vi "Verify Bitfile Selection.vi"(5 "Warning text reference":refnum<vi>, 7 "ok button reference in":refnum<vi>, 8 "error in (no error)":errorcluster, 9 "Existing RIO Device Addresses":string[](array[string]), 10 "RIO Device Address":string, 11 "file path":path) -> (0 "error out":errorcluster)   [LabVIEW 2020, in "Engine Simulation Toolkit System Explorer.lvlib"]
uses:
  Engine Simulation Toolkit System Explorer.lvlib
  Shared/Constants and GUIDs.vi
  <userlib>/_OpenG.lib/file/file.llb/File Exists - Scalar__ogtk.vi
  Shared/Engine Simulation Toolkit Shared.lvlib
panel:
  out "Valid?":bool
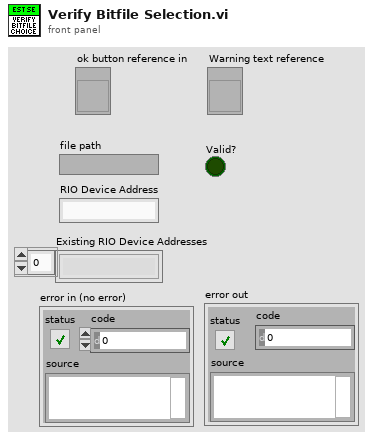
[diagram p1: front panel]
types:
  T1 = enum8{"Enabled", "Disabled", "Disabled and Grayed Out"}
  T2 = cluster{bool, "Constant.Nonexistent File":string}
  T3 = cluster{bool, "Constant.Device Address Already Exists":string}
  T4 = typedef "Engine Simulation Toolkit Shared.lvlib/Bitfile EST Version.ctl" = enum16{"1.0", "1.1", "1.2", "1.3", "1.4"}
  T5 = cluster{bool, "Constant.Multi FPGA Not Supported":string}
  T6 = cluster{bool, "Constant.Device Address Already Exists":string}[]
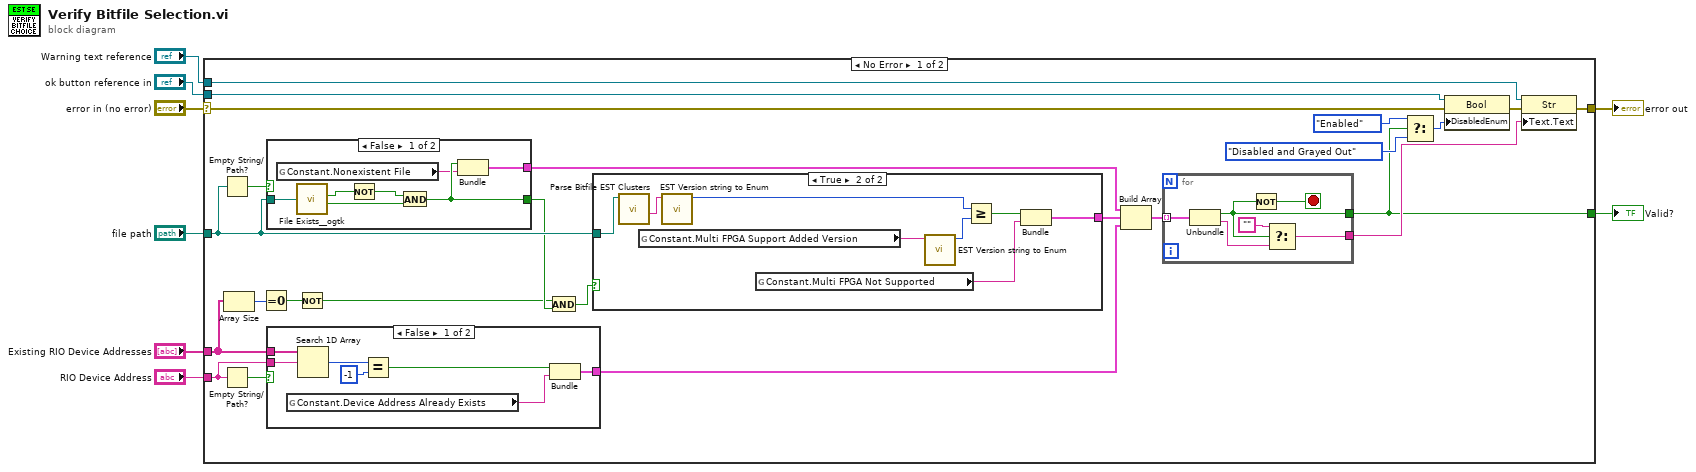
[diagram p0: block diagram]
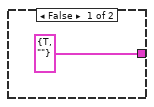
[diagram p2: hidden frame]
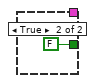
[diagram p4: hidden frame]
diagram:
  n1 = case shown="No Error" "error in (no error)" {
    selector: "error in (no error)" -> [w17 w63]
    tunnel: "ok button reference in" -> [w29 _]
    tunnel: "file path" -> [w18 _]
    tunnel: "RIO Device Address" -> [w25 _]
    tunnel: [w27 w63] -> w4
    tunnel: "Warning text reference" -> [w26 _]
    tunnel: "Existing RIO Device Addresses" -> [w21 _]
    tunnel: [w10 _] -> w1
    frame No Error {
      n2 = Empty String/Path?(string/path=w18) -> (empty?=w24:bool)
      n3 = Empty String/Path?(string/path=w25) -> (empty?=w23:bool)
      n4 = Array Size(array=w21) -> (size(s)=w22:i32)
      n5 = Equal To 0?(x=w22) -> (x = 0?=w20:bool)
      n6 = case shown="False" w24 {
        tunnel: w18 -> [w52 _]
        tunnel: [w51 FALSE] -> w11
        tunnel: [w50 _] -> w15
        frame False {
          n7 = global read "Constants and GUIDs.vi" "Constant.Nonexistent File"() -> (w49:string)
          n8 = call-poly <userlib>:"File Exists__ogtk.vi"("file path"=w52) -> ("is directory"=w55:bool, "exists"=w53:bool)  [unwired: 6 in]
          n9 = Not(x=w55) -> (.not. x?=w54:bool)
          n10 = And(x=w54, y=w53) -> (x .and. y?=w51:bool)
          n11 = Bundle(w51, "Constant.Nonexistent File"=w49) -> (w50:T2)  [unwired: 1 in]
        }
        frame True {
        }
      }
      n12 = case shown="False" w23 {
        tunnel: w25 -> [w46 _]
        tunnel: w21 -> [w45 _]
        tunnel: [w43 _] -> w14
        frame False {
          n13 = global read "Constants and GUIDs.vi" "Constant.Device Address Already Exists"() -> (w42:string)
          n14 = Search 1D Array(1D array=w45, element=w46) -> (index of element=w48:i32)  [unwired: 1 in]
          n15 = Equal?(x=w48, y=-1) -> (x = y?=w44:bool)
          n16 = Bundle(w44, "Constant.Device Address Already Exists"=w42) -> (w43:T3)  [unwired: 1 in]
        }
        frame True {
        }
      }
      n17 = Not(x=w20) -> (.not. x?=w9:bool)
      n18 = And(x=w9, y=w11) -> (x .and. y?=w19:bool)
      n19 = case shown="True" w19 {
        tunnel: w18 -> [_ w41]
        tunnel: [cluster{bool, string} {TRUE, ""} w37] -> w16
        frame False {
        }
        frame True {
          n20 = call "Parse Bitfile EST Clusters.vi"("bitfile path"=w41) -> ("version"=w39:string)  [unwired: 6 in, 4 out]
          n21 = global read "Constants and GUIDs.vi" "Constant.Multi FPGA Support Added Version"() -> (w35:string)
          n22 = call "EST Version string to Enum.vi"("EST version string"=w39) -> ("EST version enum"=w40:T4)  [unwired: 9 in, 1 out]
          n23 = global read "Constants and GUIDs.vi" "Constant.Multi FPGA Not Supported"() -> (w36:string)
          n24 = call "EST Version string to Enum.vi"("EST version string"=w35) -> ("EST version enum"=w34:T4)  [unwired: 9 in, 1 out]
          n25 = Greater Or Equal?(x=w40, y=w34) -> (x >= y?=w38:bool)
          n26 = Bundle(w38, "Constant.Multi FPGA Not Supported"=w36) -> (w37:T5)  [unwired: 1 in]
        }
      }
      n27 = Build Array(w15, w16, w14) -> (w13:T6)
      n28 = for {
        tunnel: w13 -> [w62] mode=indexing
        tunnel: [w60] -> w10
        tunnel: [w58] -> w12
        stop <- w61 stop-if-true
        n29 = Unbundle(w62) -> (w60:bool, "Constant.Device Address Already Exists"=w59:string)
        n30 = Not(x=w60) -> (.not. x?=w61:bool)
        n31 = Select(t="", s=w60, f=w59) -> (s? t:f=w58:string)
      }
      n32 = Select(t=T1."Enabled" ("Disabled"), s=w10, f=T1."Disabled and Grayed Out" ("Disabled")) -> (s? t:f=w30:T1)
      n33 = property class="Bool"(reference=w29, error in=w17, "DisabledEnum"=w30) -> (error out=w28:errorcluster)  [unwired: 1 out]
      n34 = property class="Str"(reference=w26, error in=w28, "Text.Text"=w12) -> (error out=w27:errorcluster)  [unwired: 1 out]
    }
    frame Error {
    }
  }
  "error out" <- w4
  "Valid?" <- w1
